vi "Get Named Range Values (VAR).vi"(8 "error in":errorcluster, 9 "Sheet Name":string, 10 "Named Range Identifier":string, 11 "SpreadsheetDoc in":refnum<k24>) -> (0 "error out":errorcluster, 2 "Cells":variant[][](array[variant]), 3 "SpreadsheetDoc out":refnum<k24>)   [LabVIEW 2019, in "Open Xml.lvlib"]
uses:
  Open Xml.lvlib
  D:/git/Open-Xml-LabVIEW/Source/DocumentFormat.OpenXml.dll
  DocumentFormat.OpenXml.dll
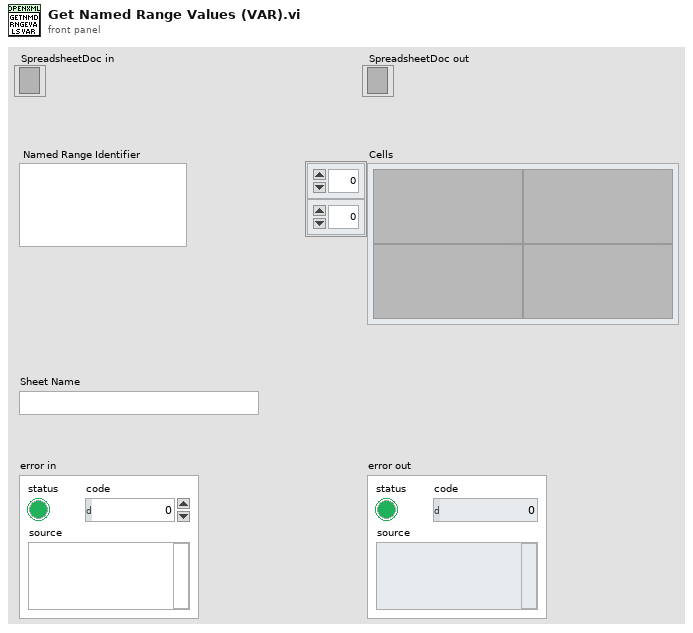
[diagram p1: front panel]
types:
  T1 = typedef "Open Xml.lvlib/Cell DataType.ctl" = enum16{"Void", "Boolean", "Number", "Error", "SharedString", "String", "InlineString", "Date"}
  T2 = cluster{"Number":dbl, "String":string, "Boolean":bool, "Time Stamp":timestamp, "Error":errorcluster}[][]
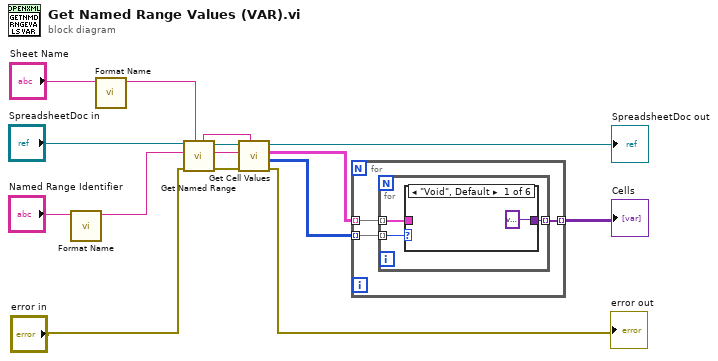
[diagram p0: block diagram]
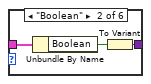
[diagram p2: hidden frame]
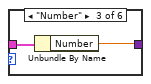
[diagram p3: hidden frame]
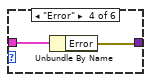
[diagram p4: hidden frame]
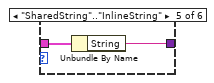
[diagram p5: hidden frame]
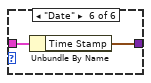
[diagram p6: hidden frame]
diagram:
  n1 = call "Format Name.vi"("Sheet Name"="Named Range Identifier") -> ("Formatted Sheet Name"=w1:string)  [unwired: 10 in]
  n2 = call "Format Name.vi"("Sheet Name"="Sheet Name") -> ("Formatted Sheet Name"=w2:string)  [unwired: 10 in]
  n3 = call "Get Named Range.vi"("Sheet Name"=w2, "error in"="error in", "Range Identifier"=w1, "SpreadsheetDoc in"="SpreadsheetDoc in") -> ("error out"=w12:errorcluster, "Range"=w9:string, "SpreadsheetDoc out"=w11:refnum<k24>, "Sheet Name"=w10:string)  [unwired: 4 in]
  n4 = call "Get Cell Values.vi"("Sheet Name"=w10, "error in"=w12, "Cell Addresses"=w9, "SpreadsheetDoc in"=w11) -> ("error out"=→"error out":errorcluster, "Types"=w6:T1[][], "Cell Values"=w8:T2, "SpreadsheetDoc out"=→"SpreadsheetDoc out":refnum<k24>)  [unwired: 4 in]
  n5 = for {
    tunnel: w8 -> [w18] mode=indexing
    tunnel: w6 -> [w17] mode=indexing
    tunnel: [w16] -> w5 mode=indexing
    n6 = for {
      tunnel: w18 -> [w20] mode=indexing
      tunnel: w17 -> [w21] mode=indexing
      tunnel: [w19] -> w16 mode=indexing
      n7 = case shown="\"Void\", Default" w21 {
        tunnel: w20 -> [_ w25 w27 w29 w31 w33]
        tunnel: [variant ("Variant") w23 w26 w28 w30 w32] -> w19
        frame "Void", Default {
        }
        frame "Boolean" {
          n8 = Unbundle By Name(w25) -> ("Boolean"=w24:bool)
          n9 = To Variant(anything=w24) -> (Variant=w23:variant)
        }
        frame "Number" {
          n10 = Unbundle By Name(w27) -> ("Number"=w26:dbl)
        }
        frame "Error" {
          n11 = Unbundle By Name(w29) -> ("Error"=w28:errorcluster)
        }
        frame "SharedString".."InlineString" {
          n12 = Unbundle By Name(w31) -> ("String"=w30:string)
        }
        frame "Date" {
          n13 = Unbundle By Name(w33) -> ("Time Stamp"=w32:timestamp)
        }
      }
    }
  }
  "Cells" <- w5
